vi "Get Device Info.vi"(8 "error in (no error)":errorcluster) -> (0 "error out":errorcluster, 2 "Kinect Properties":T1(array[cluster]), 3 "Number of Kinects Attached":i32)   [LabVIEW 2014, in "Kinect Library.lvlib"]
doc: "This VI returns an array of information about all Kinect sensors attached to this computer. This information can be used to decide which Kinect to interface with using the Initialize Kinect VI."
uses:
  Kinect Library.lvlib
  Microsoft.Kinect
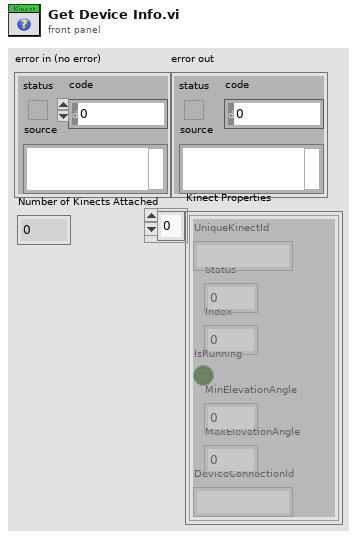
[diagram p1: front panel]
types:
  T1 = cluster{"UniqueKinectId":string, "Status":i32, "Index":i32, "IsRunning":bool, "MinElevationAngle":i32, "MaxElevationAngle":i32, "DeviceConnectionId":string}[]
  T2 = cluster{"UniqueKinectId":string, "Status":i32, "Index":i32, "IsRunning":bool, "MinElevationAngle":i32, "MaxElevationAngle":i32, "DeviceConnectionId":string}
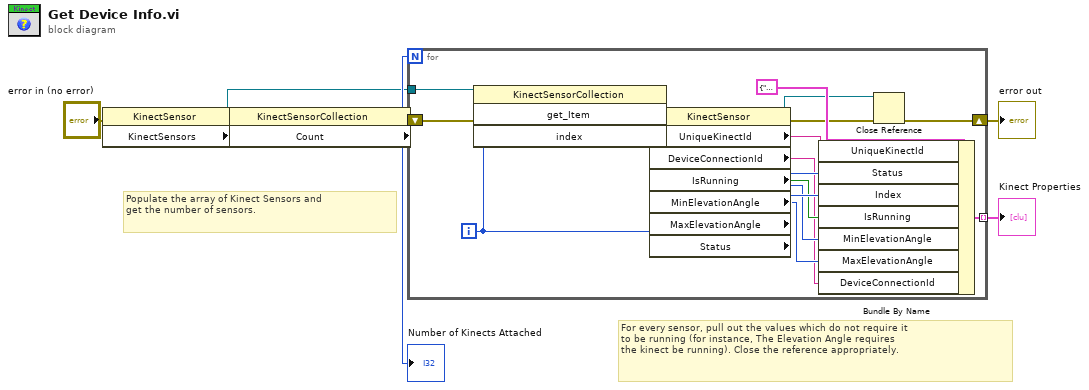
[diagram p0: block diagram]
diagram:
  # "For every sensor, pull out the values which do not require it\nto be running (for instance, The Elevation Angle requires\nthe kinect be running). Close the reference appropriately."
  # "Populate the array of Kinect Sensors and\nget the number of sensors."
  n1 = property class="KinectSensor"(error in="error in (no error)") -> (error out=w6:errorcluster, "KinectSensors"=w4:refnum<k24>)  [unwired: 1 in, 1 out]
  n2 = property class="KinectSensorCollection"(reference=w4, error in=w6) -> (error out=w3:errorcluster, "Count"=w5:i32)  [unwired: 1 out]
  "Number of Kinects Attached" <- w5
  n3 = for {
    N: w5 -> [_]
    tunnel: w4 -> [w22]
    tunnel: [w14] -> w1 mode=indexing
    shift-right: [w10] -> w2
    shift-left: w3 -> [w13]
    i -> [w20]
    n4 = invoke class="KinectSensorCollection" method="get_Item"(reference=w22, error in=w13, "index"=w20) -> ("get_Item"=w9:refnum<k24>)  [unwired: 1 in, 3 out]
    n5 = property class="KinectSensor"(reference=w9) -> (reference out=w11:refnum<k24>, error out=w12:errorcluster, "UniqueKinectId"=w19:string, "DeviceConnectionId"=w8:string, "IsRunning"=w17:bool, "MinElevationAngle"=w16:i32, "MaxElevationAngle"=w15:i32, "Status"=w18:i32)  [unwired: 1 in]
    n6 = Bundle By Name(cluster=T2 {"UniqueKinectId"="", "Status"=0, "Index"=0, "IsRunning"=FALSE, "MinElevationAngle"=0, "MaxElevationAngle"=0, "DeviceConnectionId"=""}, "UniqueKinectId"=w19, "Status"=w18, "Index"=w20, "IsRunning"=w17, "MinElevationAngle"=w16, "MaxElevationAngle"=w15, "DeviceConnectionId"=w8) -> (w14:T2)
    n7 = Close Reference(reference=w11, error in (no error)=w12) -> (error out=w10:errorcluster)
  }
  "error out" <- w2
  "Kinect Properties" <- w1
